vi "Analog Read Pin.vi"(8 "Error In":errorcluster, 10 "Analog Pin":T1, 11 "ChipKit Resource":T2={"COM Port"="COM3", "Board Type"=enum."ChipKit uC32", "Connection Type"=enum."USB / Serial", "Baud Rate (115200)"=15, "Bytes Per Packet (15)"=15}) -> (0 "Error Out":errorcluster, 2 "Voltage":dbl, 3 "ChipKit Resource":T2={"COM Port"="COM11", "Board Type"=enum."ChipKit uC32", "Connection Type"=enum."USB / Serial", "Baud Rate (115200)"=15, "Bytes Per Packet (15)"=15})   [LabVIEW 2011, in "LabVIEW Interface for ChipKit.lvlib"]
doc: "Reads the analog voltage on the selected ChipKit analog input pin.\nNote: Chipkit jumpers JP6 and JP8 must be set to A4 and A5 respectivly to use analog inputs 4 and 5."
uses:
  LabVIEW Interface for ChipKit.lvlib
  Private/Type Defs/Chipkit Resource.ctl
  Private/Type Defs/Board Type.ctl
  Private/Type Defs/Connection Type.ctl
  Private/Type Defs/Analog Pin.ctl
  Private/Type Defs/Command.ctl
  Private/Type Defs/Pin Type.ctl
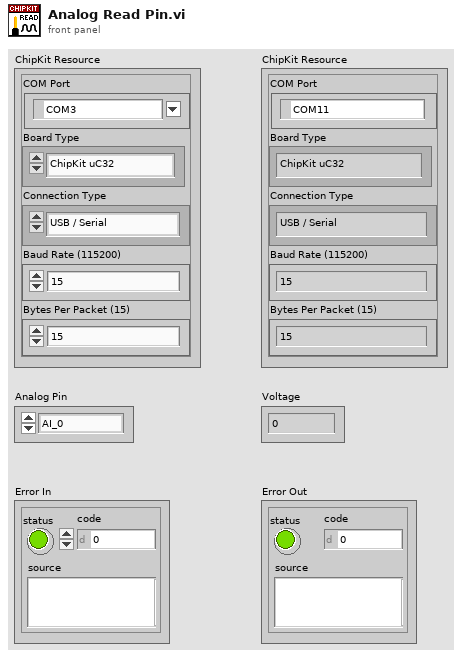
[diagram p1: front panel]
types:
  T1 = typedef "LabVIEW Interface for ChipKit.lvlib/Analog Pin.ctl" = enum16{"AI_0", "AI_1", "AI_2", "AI_3", "AI_4", "AI_5", "AI_6", "AI_7", "AI_8", "AI_9", "AI_10", "AI_11", "AI_12", "AI_13", "AI_14", "AI_15"}
  T2 = typedef "LabVIEW Interface for ChipKit.lvlib/Chipkit Resource.ctl" = cluster{"COM Port":refnum<visa-resource-name>, "Board Type":T3, "Connection Type":T4, "Baud Rate (115200)":u32, "Bytes Per Packet (15)":u32}
  T3 = typedef "LabVIEW Interface for ChipKit.lvlib/Board Type.ctl" = enum16{"ChipKit uC32", "ChipKit Uno32", "ChipKit Max32"}
  T4 = typedef "LabVIEW Interface for ChipKit.lvlib/Connection Type.ctl" = enum8{"USB / Serial", "XBEE", "BlueSmirf (Bluetooth)"}
  T5 = typedef "LabVIEW Interface for ChipKit.lvlib/Pin Type.ctl" = enum8{"Analog", "Digital", "PWM", "Tone"}
  T6 = typedef "LabVIEW Interface for ChipKit.lvlib/Command.ctl" = enum8{"setArduinoMode", "flushSerial", "setPinMode", "digitalWritePin", "digitalWritePort", "tone", "digitalReadPin", "digitalReadPort", "analogReadPin", "analogReadPort", "pwmWritePin", "pwmWritePort", "sevenSegment_Configure", "sevenSegment_Write", "I2C Init", "I2C Write", "I2C Read", "SPI Init", "SPI Set Bit Order", "SPI Set Clock Divider", "SPI Set Data Mode", "SPI Send / Receive", "SPI Close", "Servo Set Num Servos", "Servo Config Servo", "Servo Write Angle", "Servo Read Angle", "Servo Write Pulse Width", "Servo Read Pulse Width", "Servo Detach", "LCD Init", "LCD Set Size", "LCD Set Cursor Mode", "LCD Clear", "LCD Set Cursor Position", "LCD Print", "LCD Display Power", "LCD Scroll Display", "LCD Autoscroll", "LCD Print Direction", "LCD Create Custom Char", "LCD Print Custom Char", "contAcqOn", "contAcqOff", "getFirmwareVersion", "FiniteSampleStart", "NA", "NA2", "Conifg Stepper", "Stepper Write", "Stepper Detach", "Stepper Steps To Go", "Config DO Port", "Config DI Port"}
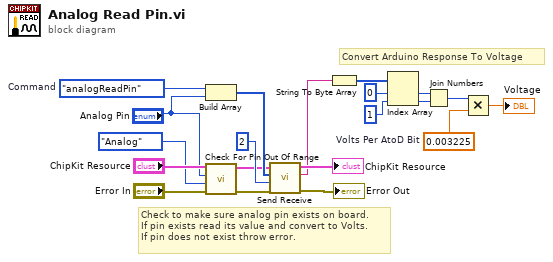
[diagram p0: block diagram]
diagram:
  w17 = 0.003225  # Volts Per AtoD Bit
  w15 = Command."analogReadPin"  # Command
  # "Check to make sure analog pin exists on board.\nIf pin exists read its value and convert to Volts.\nIf pin does not exist throw error."
  # "Convert Arduino Response To Voltage"
  n1 = Build Array(w15, "Analog Pin") -> (w14:u16[])
  n2 = call "Check For Pin Out Of Range.vi"("Error In"="Error In", "Pin Type"=Pin_Type."Analog", "User Pin Number"="Analog Pin", "Arduino Resource"="ChipKit Resource") -> ("Error Out"=w8:errorcluster, "Arduino Resource"=w6:T2)  [unwired: 6 in]
  n3 = call "Send Receive.vi"("Error In"=w8, "Bytes To Read (0)"=u32 2, "Data"=w14, "ChipKit Resource"=w6) -> ("Error Out"=→"Error Out":errorcluster, "Read Buffer"=w10:string, "ChipKit Resource"=→"ChipKit Resource":T2)  [unwired: 5 in]
  n4 = String To Byte Array(string=w10) -> (unsigned byte array=w20:u8[])
  n5 = Index Array(array=w20, index #1=0 ("index"), index #2=1 ("index")) -> (element #1=w5:u8, element #2=w4:u8)
  n6 = Join Numbers(hi=w5, lo=w4) -> ((hi.lo)=w3:u16)
  n7 = Multiply(x=w3, y=w17) -> (x*y=→"Voltage":dbl)
